vi "Scan Initilize_ver2.vi"(4 "Enable DMM Relay":bool=TRUE, 6 "Measure Maximun Voltage":dbl=100.0 format="%#_13g", 7 "Scan Measure\nTime":dbl=17.0, 8 "error in (no error)":errorcluster, 9 "Current Setting":u8[](array[numeric]), 10 "Channel Count":i32, 11 "VISA Refnum in":refnum<visa-resource-name>) -> (0 "error out":errorcluster, 1 "N channel number":i32, 2 "P channel number":i32, 3 "VISA Refnum out":refnum<visa-resource-name>, 5 "Current Channel":string[](array[string]))   [LabVIEW 2023]
uses:
  <instrlib>/Agilent 3446X Series/Agilent 3446X Series.lvlib
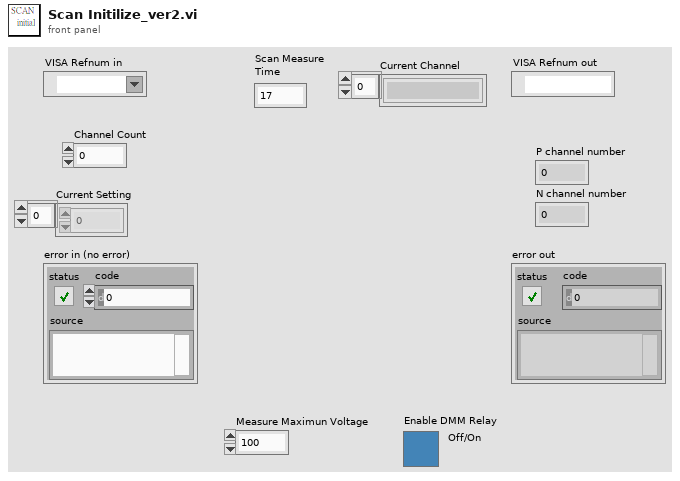
[diagram p1: front panel]
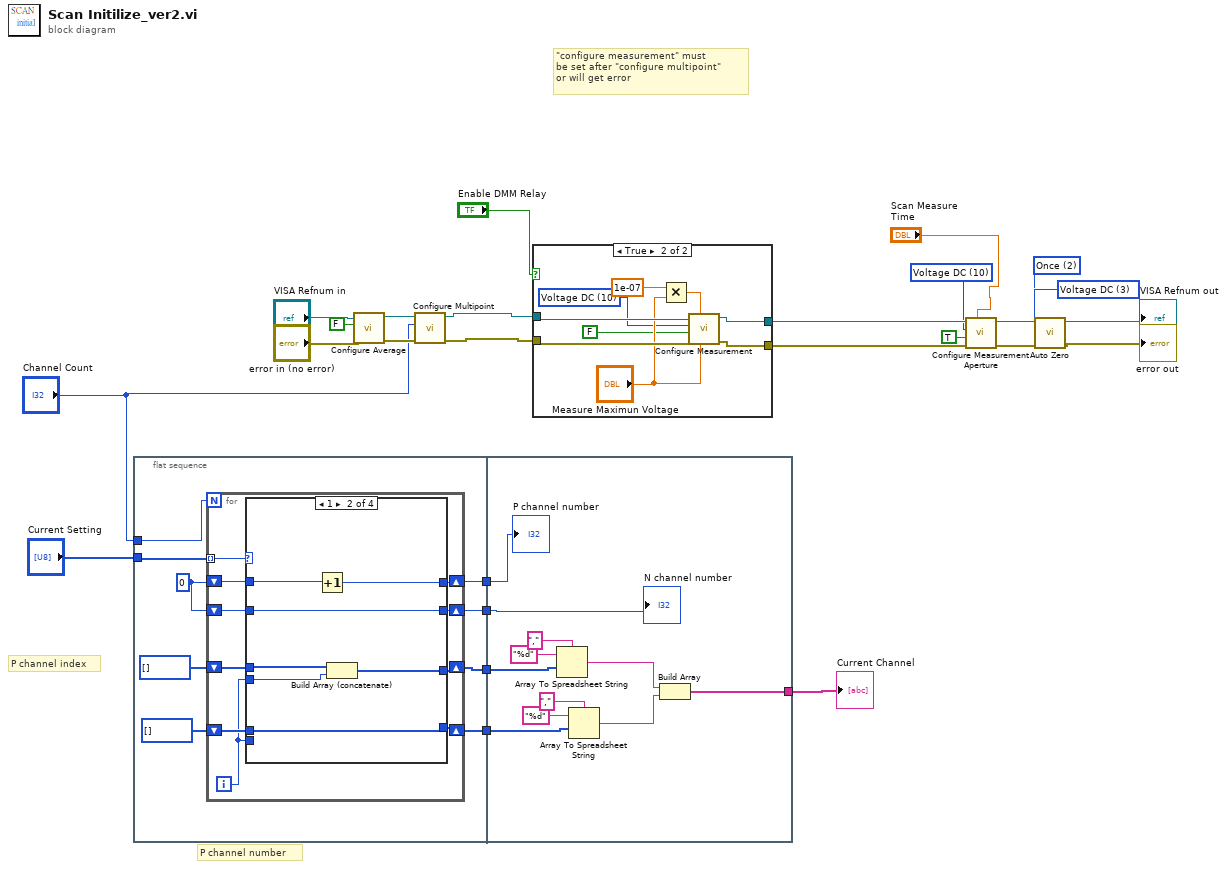
[diagram p0: block diagram]
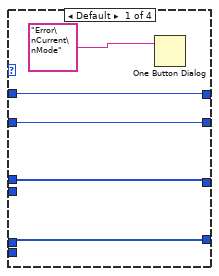
[diagram p3: hidden frame]
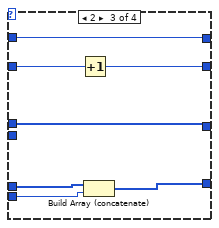
[diagram p4: hidden frame]
diagram:
  w13 = 3 items=["Current DC", "Resistance", "Temperature", "Voltage DC"] ("Zero Type (0: Current DC)")
  w12 = 2 items=["Disable", "Enable", "Once"] ("Auto Zero (1: Enable)")
  w10 = 10 items=["Continuity", "Current AC", "Current DC", "Diode", "Frequency", "Resistance 4-wire", "Period", "Resistance 2-wire", "Temperature", "Voltage AC", "Voltage DC", "Voltage DC Ratio", "Capacitance"] ("Measurement Function (0: Continuity)")
  # "P channel index"
  # "P channel number"
  # "\"configure measurement\" must \nbe set after \"configure multipoint\"\nor will get error"
  n1 = flat-sequence {
    tunnel: "Channel Count" -> [w35]
    tunnel: "Current Setting" -> [w34]
    tunnel: [w32] -> w8
    tunnel: [w31] -> w7
    tunnel: [w28] -> w4
    tunnel: [w27] -> w3
    tunnel: w8 -> [w79]
    tunnel: w7 -> [w78]
    tunnel: w4 -> [w75]
    tunnel: w3 -> [w72]
    tunnel: [w69] -> w2
    frame #0 {
      w33 = 0 ("P_current_count")
      n2 = for {
        N: w35 -> [_]
        tunnel: w34 -> [w45] mode=indexing
        shift-right: [w43] -> w32
        shift-left: w33 -> [w44]
        shift-right: [w41] -> w31
        shift-left: w33 -> [w42]
        shift-right: [w39] -> w28
        shift-left: i32[] [] -> [w40]
        shift-right: [w37] -> w27
        shift-left: i32[] [] -> [w38]
        i -> [w36]
        n3 = case shown="1" w45 {
          tunnel: w44 -> [w49 w57 w62 w68]
          tunnel: [w49 w56 w62 w68] -> w43
          tunnel: w42 -> [w48 w55 w64 w67]
          tunnel: [w48 w55 w63 w67] -> w41
          tunnel: w40 -> [w46 w54 w58 w66]
          tunnel: w36 -> [_ w53 _ _]
          tunnel: [w46 w52 w58 w66] -> w39
          tunnel: w38 -> [w47 w51 w61 w65]
          tunnel: [w47 w51 w60 w65] -> w37
          tunnel: w36 -> [_ _ w59 _]
          frame Default {
            n4 = One Button Dialog(message="Error\nCurrent\nMode" ("error source (\" \")")) -> ()  [unwired: 1 in, 1 out]
          }
          frame 1 {
            n5 = Increment(x=w57) -> (x+1=w56:i32)
            n6 = Build Array (concatenate)(w54, w53) -> (w52:i32[])
          }
          frame 2 {
            n7 = Increment(x=w64) -> (x+1=w63:i32)
            n8 = Build Array (concatenate)(w61, w59) -> (w60:i32[])
          }
          frame 0 {
          }
        }
      }
    }
    frame #1 {
      n9 = Array To Spreadsheet String(delimiter (Tab)=",", array=w75, 3:"%d" ("format string")) -> (spreadsheet string=w71:string)
      n10 = Array To Spreadsheet String(delimiter (Tab)=",", array=w72, 3:"%d" ("format string")) -> (spreadsheet string=w70:string)
      n11 = Build Array(w71, w70) -> (w69:string[])
      "P channel number" <- w79
      "N channel number" <- w78
    }
  }
  n12 = call <instrlib>:"Configure Average.vi"("error in (no error)"="error in (no error)", "Enable Statistics (F: Disable)"=FALSE, "VISA resource name"="VISA Refnum in") -> ("error out"=w20:errorcluster, "VISA resource name out"=w19:refnum<visa-resource-name>)  [unwired: 7 in]
  n13 = call <instrlib>:"Configure Multipoint.vi"("error in (no error)"=w20, "Trigger Count (1)"="Channel Count", "VISA resource name"=w19) -> ("error out"=w22:errorcluster, "VISA resource name out"=w21:refnum<visa-resource-name>)  [unwired: 4 in, 3 out]
  n14 = case shown="True" "Enable DMM Relay" {
    tunnel: [w80 w90] -> w24
    tunnel: [w81 w89] -> w23
    tunnel: w22 -> [w80 w88]
    tunnel: w21 -> [w81 w87]
    frame False {
    }
    frame True {
      w83 = 10 items=["Continuity", "Current AC", "Current DC", "Diode", "Frequency", "Resistance 4-wire", "Period", "Resistance 2-wire", "Temperature", "Voltage AC", "Voltage DC", "Voltage DC Ratio", "Capacitance"] ("Measurement Function (10: Voltage DC)")
      n15 = Multiply(x=1e-07, y="Measure Maximun Voltage") -> (x*y=w84:dbl)
      n16 = call <instrlib>:"Configure Measurement.vi"("Manual Range (1)"="Measure Maximun Voltage", "Absolute Resolution (1E-6)"=w84, "error in (no error)"=w88, "Auto Range (T: Enable)"=FALSE, "Measurement Function (10: Voltage DC)"=w83, "VISA resource name"=w87) -> ("error out"=w90:errorcluster, "VISA resource name out"=w89:refnum<visa-resource-name>)  [unwired: 4 out]
    }
  }
  n17 = call <instrlib>:"Configure Measurement Aperture.vi"("Aperture Time (0.1s)"="Scan Measure\nTime", "error in (no error)"=w24, "Enable Aperture (F: Disable)"=TRUE, "Measurement Function (0: Continuity)"=w10, "VISA resource name"=w23) -> ("error out"=w14:errorcluster, "VISA resource name out"=w18:refnum<visa-resource-name>)  [unwired: 5 in]
  n18 = call <instrlib>:"Auto Zero.vi"("error in (no error)"=w14, "Auto Zero (1: Enable)"=w12, "Zero Type (0: Current DC)"=w13, "VISA resource name"=w18) -> ("error out"=→"error out":errorcluster, "VISA resource name out"=→"VISA Refnum out":refnum<visa-resource-name>)  [unwired: 6 in]
  "Current Channel" <- w2
